vi "Get URL Contents.vi"(8 "error in (no error)":errorcluster, 11 "URL":string="http://macdailynews.com/index.php/weblog/rss_2.0") -> (0 "error out":errorcluster, 3 "Contents":string)   [LabVIEW 2017, in "Feed.lvclass"]
uses:
  <vilib>/NI_RSS/Feed/Feed.lvclass
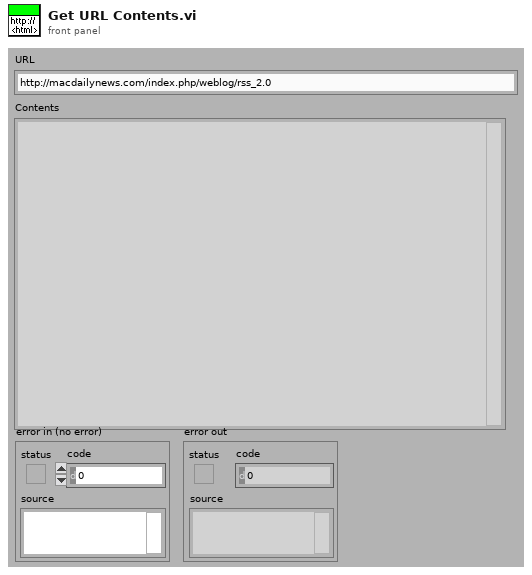
[diagram p1: front panel]
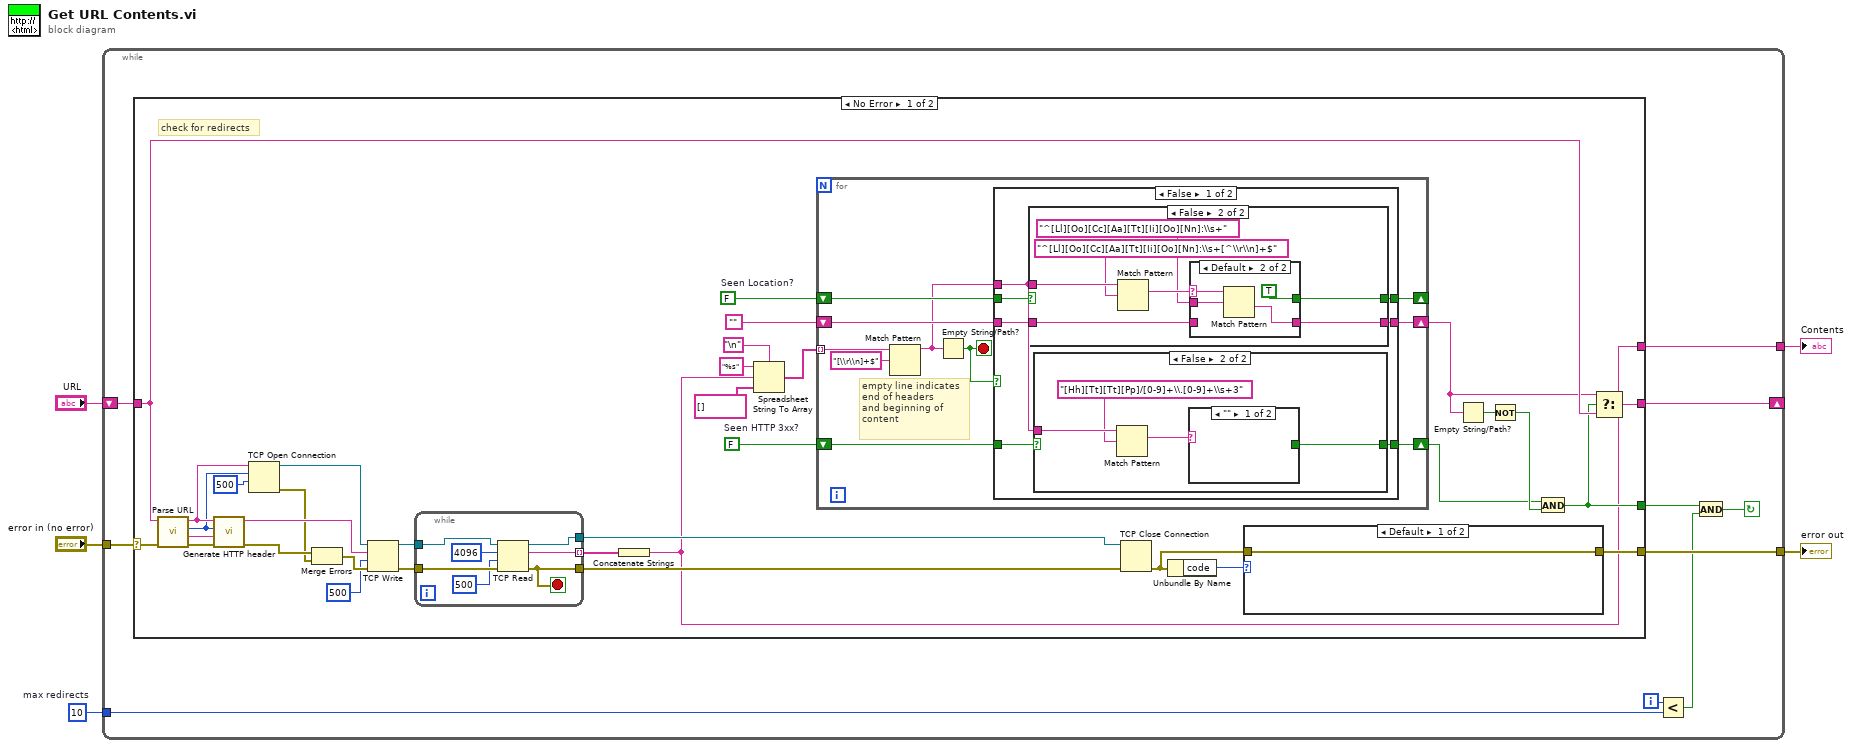
[diagram p0: block diagram]
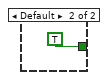
[diagram p3: hidden frame]
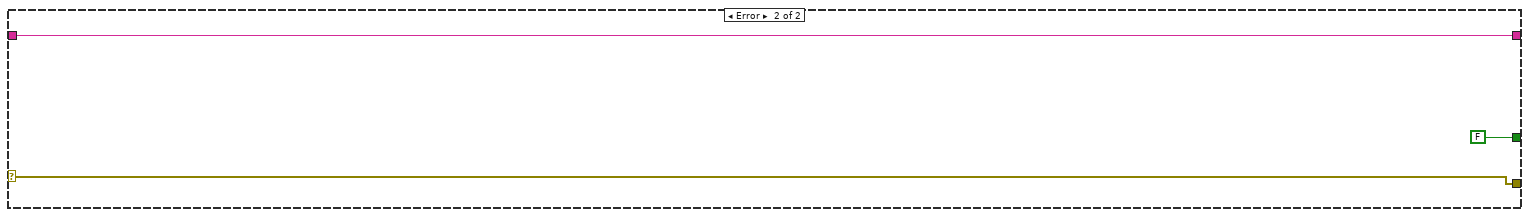
[diagram p8: hidden frame]
diagram:
  w1 = 10  # max redirects
  n1 = while {
    tunnel: [w14] -> w4
    tunnel: "error in (no error)" -> [w13]
    shift-right: [w11] -> _
    shift-left: "URL" -> [w15]
    tunnel: [w12] -> w2
    tunnel: w1 -> [w8]
    i -> [w9]
    stop <- w6 continue-if-true
    n2 = case shown="No Error" w13 {
      selector: w13 -> [w34 w101]
      tunnel: w15 -> [w30 w100]
      tunnel: [w20 _] -> w12
      tunnel: [w35 w101] -> w14
      tunnel: [w29 w100] -> w11
      tunnel: [w28 FALSE] -> w10
      frame No Error {
        w24 = FALSE  # Seen HTTP 3xx?
        w27 = FALSE  # Seen Location?
        # "check for redirects"
        n3 = call <vilib>:"Parse URL.vi"("error in (no error)"=w34, "URL"=w30) -> ("error out"=w49:errorcluster, "Path"=w50:string, "Port"=w47:i32, "Server"=w48:string)  [unwired: 6 out]
        n4 = call <vilib>:"Generate HTTP header.vi"("error out"=w49, "Path"=w50, "Port"=w47, "Server"=w48) -> ("error IO"=w44:errorcluster, "HTTP Header"=w45:string)  [unwired: 2 out]
        n5 = TCP Open Connection(address=w48, remote port or service name=w47, timeout ms (60000)=500) -> (connection ID=w46:refnum<k5>, error out=w43:errorcluster)  [unwired: 1 in, 1 out]
        n6 = Merge Errors(w44, w43) -> (w42:errorcluster)
        n7 = TCP Write(connection ID=w46, data in=w45, error in (no error)=w42, 9:500 ("timeout ms (25000)")) -> (connection ID out=w41:refnum<k5>, error out=w40:errorcluster)  [unwired: 1 out]
        n8 = while {
          tunnel: w41 -> [w98]
          tunnel: w40 -> [w97]
          tunnel: [w94] -> w21 mode=indexing
          tunnel: [w96] -> w37
          tunnel: [w95] -> w39
          stop <- w96 stop-if-true
          n9 = TCP Read(connection ID=w98, bytes to read=4096, error in (no error)=w97, 9:500 ("timeout ms (25000)")) -> (connection ID out=w95:refnum<k5>, data out=w94:string, error out=w96:errorcluster)  [unwired: 1 out]
        }
        n10 = Concatenate Strings(w21) -> (w20:string)
        n11 = Spreadsheet String To Array(delimiter (Tab)="\n", format string="%s", spreadsheet string=w20, array type (2D Dbl)=string[] []) -> (array=w22:string[])
        n12 = for {
          tunnel: w22 -> [w54] mode=indexing
          shift-right: [w57] -> _
          shift-left: w27 -> [w60]
          shift-right: [w58] -> w25
          shift-left: "" -> [w59]
          shift-right: [w55] -> w23
          shift-left: w24 -> [w56]
          stop <- w51 stop-if-true
          # "empty line indicates\nend of headers\nand beginning of\ncontent"
          n13 = Match Pattern(string=w54, regular expression="[\\r\\n]+$") -> (before substring=w52:string)  [unwired: 1 in, 3 out]
          n14 = Empty String/Path?(string/path=w52) -> (empty?=w51:bool)
          n15 = case shown="False" w51 {
            tunnel: w60 -> [w67 w89]
            tunnel: w59 -> [w66 w90]
            tunnel: [w65 w90] -> w58
            tunnel: [w64 w89] -> w57
            tunnel: w52 -> [w63 _]
            tunnel: w56 -> [w62 w88]
            tunnel: [w61 w88] -> w55
            frame False {
              n16 = case shown="False" w67 {
                selector: w67 -> [w75 _]
                tunnel: w63 -> [_ w82]
                tunnel: w66 -> [w74 w78]
                tunnel: [w74 w77] -> w65
                tunnel: [w75 w76] -> w64
                frame True {
                }
                frame False {
                  n17 = Match Pattern(string=w82, regular expression="^[Ll][Oo][Cc][Aa][Tt][Ii][Oo][Nn]:\\s+[^\\r\\n]+$") -> (match substring=w80:string)  [unwired: 1 in, 3 out]
                  n18 = case shown="Default" w80 {
                    selector: w80 -> [_ w87]
                    tunnel: [w83 w86] -> w77
                    tunnel: "^[Ll][Oo][Cc][Aa][Tt][Ii][Oo][Nn]:\\s+" ("regular expression") -> [_ w85]
                    tunnel: w78 -> [w83 _]
                    tunnel: [_ TRUE] -> w76
                    frame "" {
                    }
                    frame Default {
                      n19 = Match Pattern(string=w87, regular expression=w85) -> (after substring=w86:string)  [unwired: 1 in, 3 out]
                    }
                  }
                }
              }
              n20 = case shown="False" w62 {
                selector: w62 -> [w68 _]
                tunnel: w63 -> [_ w72]
                tunnel: [w68 w69] -> w61
                frame True {
                }
                frame False {
                  n21 = Match Pattern(string=w72, regular expression="[Hh][Tt][Tt][Pp]/[0-9]+\\.[0-9]+\\s+3") -> (match substring=w70:string)  [unwired: 1 in, 3 out]
                  n22 = case shown="\"\"" w70 {
                    tunnel: [_ TRUE] -> w69
                    frame "" {
                    }
                    frame Default {
                    }
                  }
                }
              }
            }
            frame True {
            }
          }
        }
        n23 = TCP Close Connection(connection ID=w39, error in (no error)=w37) -> (error out=w36:errorcluster)  [unwired: 2 out]
        n24 = Unbundle By Name(w36) -> ("code"=w38:i32)
        n25 = case shown="Default" w38 {
          tunnel: w36 -> [w91 _]
          tunnel: [w91 _] -> w35
          frame Default {
          }
          frame 66 {
            # "Ignore error 66 (network connection closed)\nbecause it's not a problem if we read beyond\nthe available bytes."
          }
        }
        n26 = Empty String/Path?(string/path=w25) -> (empty?=w32:bool)
        n27 = Not(x=w32) -> (.not. x?=w31:bool)
        n28 = And(x=w23, y=w31) -> (x .and. y?=w28:bool)
        n29 = Select(t=w25, s=w28, f=w30) -> (s? t:f=w29:string)
      }
      frame Error {
      }
    }
    n30 = Less?(x=w9, y=w8) -> (x < y?=w7:bool)
    n31 = And(x=w10, y=w7) -> (x .and. y?=w6:bool)
  }
  "Contents" <- w2
  "error out" <- w4
